vi "Save_Trav_setup.vi"(0 "Work in Tunnel Coordinates?":T1, 1 "Trav Table":T2[](array[typedef]) {"Row Duration (mins)" format="%#.1f"; "Row No" min=0; "Trace Gas Concentration (%)" min=0.0 format="%#.2f"; "Emission Rate (l/min)" format="%#.2f"; "Tunnel Speed" format="%#.2f"; "Start X" format="%#.2f"; "Start Y" format="%#.2f"; "Start Z" format="%#.2f"; "End X" format="%#.2f"; "End Y" format="%#.2f"; "End Z" format="%#.2f"; "Averaging time (min)" min=0.0 format="%#.1f"}, 3 "Jump Bad Positions":bool, 4 "Setup filename":path) -> (5 "Trav Table Out":T2[](array[typedef]) {"Row Duration (mins)" format="%#.1f"; "Row No" min=0; "Trace Gas Concentration (%)" min=0.0 format="%#.2f"; "Emission Rate (l/min)" format="%#.2f"; "Tunnel Speed" format="%#.2f"; "Start X" format="%#.2f"; "Start Y" format="%#.2f"; "Start Z" format="%#.2f"; "End X" format="%#.2f"; "End Y" format="%#.2f"; "End Z" format="%#.2f"; "Averaging time (min)" min=0.0 format="%#.1f"})   [LabVIEW 2010]
uses:
  Traverse_cluster.ctl
  Spacing.ctl
  Controls/Multi_run_mode.ctl
  Controls/Tunnel_Coordinates.ctl
  Globals/Constants_global.vi
panel:
  # "X           Y            Z"
  # "Start"
  # "End"
  # "X           Y            Z"
  # "Start"
  # "End"
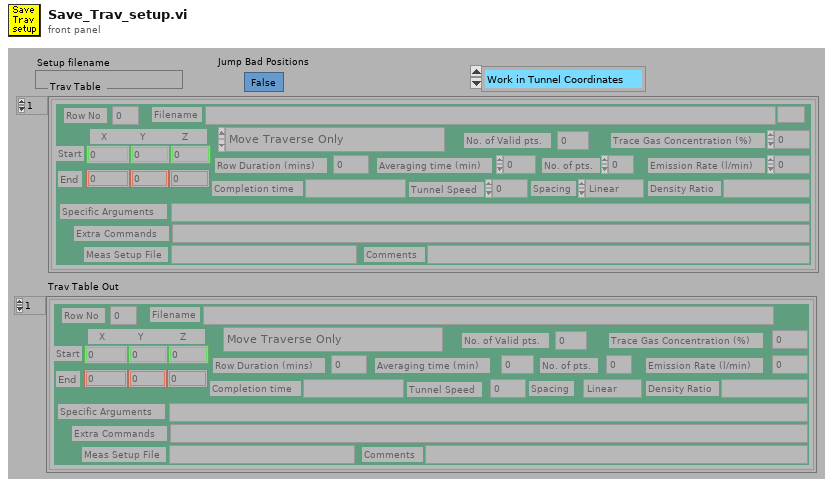
[diagram p1: front panel]
types:
  T1 = typedef "Tunnel_Coordinates.ctl" = enum16{"Work in Tunnel Coordinates", "Work in Model Coordinates"}
  T2 = typedef "Traverse_cluster.ctl" = cluster{"Start X":dbl, "Start Y":dbl, "Start Z":dbl, "End X":dbl, "End Y":dbl, "End Z":dbl, "No. of pts.":i32, "Spacing":T3, "Filename":path, "Tunnel Speed":dbl, "Averaging time (min)":dbl, "Extra Commands":string, "Specific Arguments":string, "Emission Rate (l/min)":dbl, "Trace Gas Concentration (%)":dbl, "Density Ratio":string, "Comments":string, "Row No":i32, "Row Type Selector":T4, "Completion time":string, "Row Duration (mins)":dbl, "No. of Valid pts.":i32, "Meas Setup File":string}
  T3 = typedef "Spacing.ctl" = enum16{"Linear", "Log", "Gauss", "Specified", "N/A"}
  T4 = typedef "Multi_run_mode.ctl" = enum16{"Move Traverse Only", "Set Tunnel Speed Only", "Set Source Only", "Set Measurement Conditions", "Single Measurement", "Vertical Profile", "Lateral Profile", "Longitudinal Profile", "Explore Volume", "Multi-Axis Profile", "Auto Calibrate", "Meas Fast FID Bkgnd", "Check Beam Power", "Scanning Valve Measurement", "Run VI Named:", "Set ADAM Ch", "Wait (minutes)", "Send Message", "Synchronize With:", "Fall Back to this Row", "Turn Off Row Repeating", "Blank Row"}
  T5 = enum16{"All Channel Names", "Valid Channel Names"}
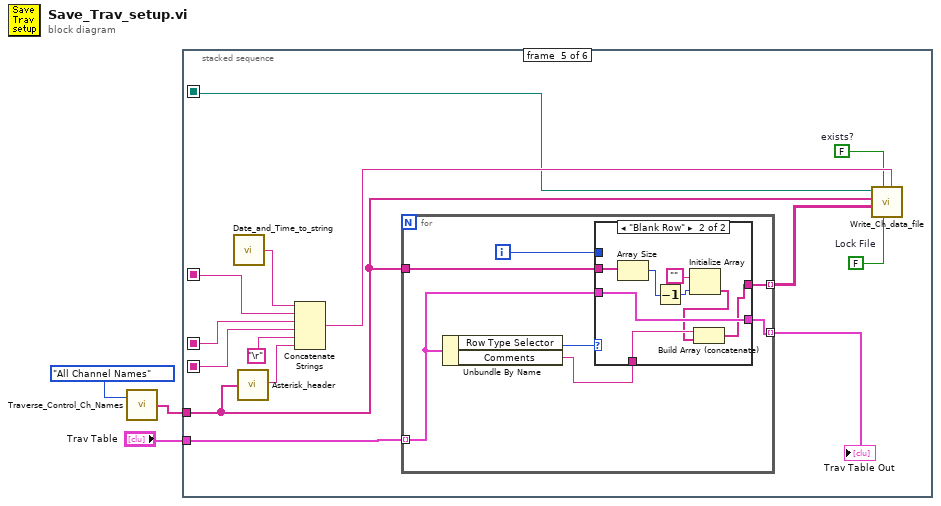
[diagram p0: block diagram]
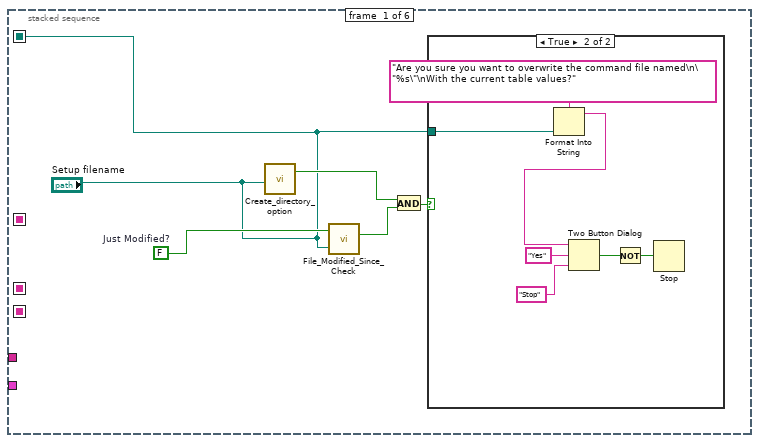
[diagram p2: hidden frame]
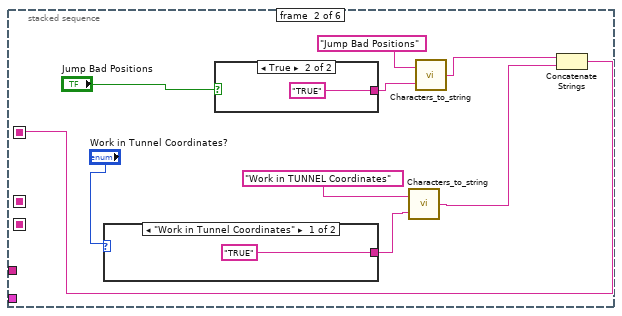
[diagram p4: hidden frame]
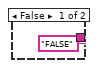
[diagram p5: hidden frame]
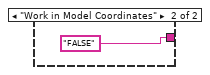
[diagram p6: hidden frame]
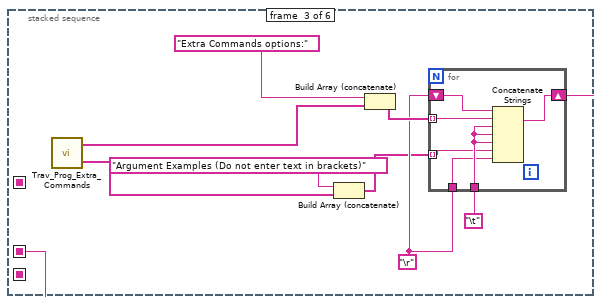
[diagram p7: hidden frame]
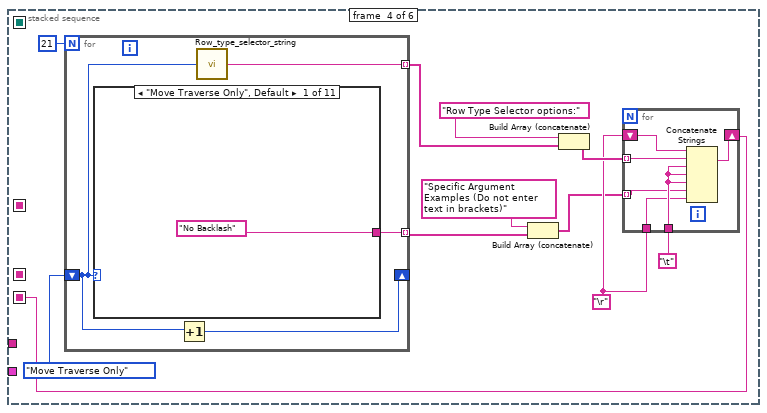
[diagram p8: hidden frame]
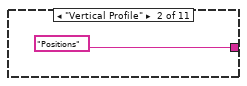
[diagram p9: hidden frame]
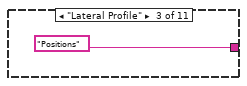
[diagram p10: hidden frame]
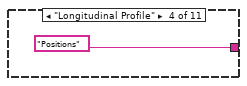
[diagram p11: hidden frame]
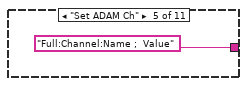
[diagram p12: hidden frame]
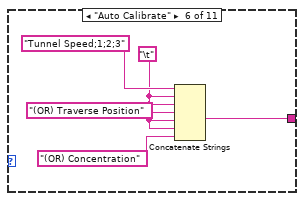
[diagram p13: hidden frame]
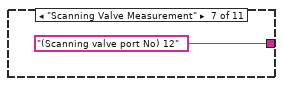
[diagram p14: hidden frame]
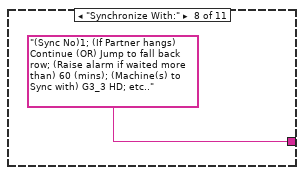
[diagram p15: hidden frame]
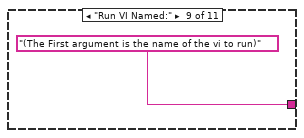
[diagram p16: hidden frame]
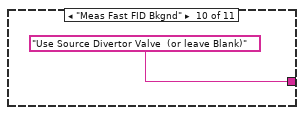
[diagram p17: hidden frame]
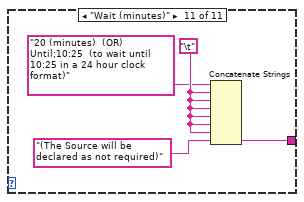
[diagram p18: hidden frame]
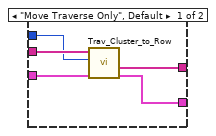
[diagram p19: hidden frame]
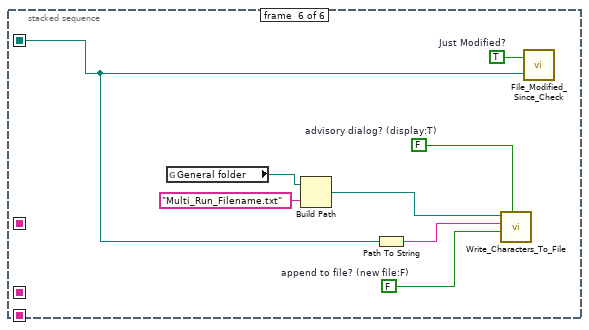
[diagram p20: hidden frame]
diagram:
  n1 = call "Traverse_Control_Ch_Names.vi"("Mode"=T5."All Channel Names") -> ("Channel names"=w3:string[])  [unwired: 1 in]
  n2 = stacked-sequence {
    seq-local: [_ w24 _ _ _ _] -> [_ _ _ _ w92 _]
    seq-local: [_ _ w35 _ _ _] -> [_ _ _ _ w94 _]
    seq-local: [_ _ _ w48 _ _] -> [_ _ _ _ w91 _]
    seq-local: ["Setup filename" _ _ _ _ _] -> [_ _ _ _ w84 w120]
    tunnel: w3 -> [_ _ _ _ w90 _]
    tunnel: "Trav Table" -> [_ _ _ _ w83 _]
    frame #0 {
      w5 = FALSE  # Just Modified?
      n3 = call "Create_directory_option.vi"("Filename"="Setup filename") -> ("Path is to existing File"=w7:bool)  [unwired: 1 out]
      n4 = call "File_Modified_Since_Check.vi"("Pathname"="Setup filename", "Just Modified?"=w5) -> ("Modified?"=w8:bool)
      n5 = And(x=w7, y=w8) -> (x .and. y?=w6:bool)
      n6 = case shown="True" w6 {
        tunnel: "Setup filename" -> [_ w15]
        frame False {
        }
        frame True {
          n7 = Format Into String(format string="Are you sure you want to overwrite the command file named\n\"%s\"\nWith the current table values?" ("Format String"), w15) -> (resulting string=w13:string)  [unwired: 2 in, 1 out]
          n8 = Two Button Dialog(message=w13, 1:"Stop" ("F button name (\"Cancel\")"), 2:"Yes" ("T button name (\"OK\")")) -> (T button?=w10:bool)
          n9 = Not(x=w10) -> (.not. x?=w9:bool)
          n10 = Stop(stop? (T)=w9) -> ()
        }
      }
    }
    frame #1 {
      n11 = case shown="\"Work in Tunnel Coordinates\"" "Work in Tunnel Coordinates?" {
        tunnel: ["TRUE" "FALSE" ("f")] -> w20
        frame "Work in Tunnel Coordinates" {
        }
        frame "Work in Model Coordinates" {
        }
      }
      n12 = case shown="True" "Jump Bad Positions" {
        tunnel: ["FALSE" ("f") "TRUE"] -> w18
        frame False {
        }
        frame True {
        }
      }
      n13 = call "Characters_to_string.vi"("Characters to write"=w20, "Label for characters"="Work in TUNNEL Coordinates") -> ("Output string"=w22:string)
      n14 = call "Characters_to_string.vi"("Characters to write"=w18, "Label for characters"="Jump Bad Positions") -> ("Output string"=w16:string)
      n15 = Concatenate Strings(w16, w22) -> (w24:string)
    }
    frame #2 {
      w36 = "\r"
      n16 = call "Trav_Prog_Extra_Commands.vi"() -> ("Extra Commands Array"=w33:string[], "Argument Examples"=w32:string[])  [unwired: 1 out]
      n17 = Build Array (concatenate)("Argument Examples (Do not enter text in brackets)" ("Substring"), w32) -> (w31:string[])
      n18 = Build Array (concatenate)("Extra Commands options:", w33) -> (w37:string[])
      n19 = for {
        shift-right: [w41] -> w35
        shift-left: w36 -> [w42]
        tunnel: w37 -> [w43] mode=indexing
        tunnel: w36 -> [w38]
        tunnel: w31 -> [w39] mode=indexing
        tunnel: "\t" -> [w40]
        n20 = Concatenate Strings(w42, w43, w40, w40, w40, w39, w38) -> (w41:string)
      }
    }
    frame #3 {
      w53 = "\r"
      n21 = for {
        N: 21 -> [_]
        shift-right: [w58] -> _
        shift-left: Multi_run_mode."Move Traverse Only" ("Mode") -> [w57]
        tunnel: [w56] -> w46 mode=indexing
        tunnel: [w55] -> w45 mode=indexing
        n22 = case shown="\"Move Traverse Only\", Default" w57 {
          tunnel: ["No Backlash" "Positions" "Positions" "Positions" "Full:Channel:Name ;  Value" w68 "(Scanning valve port No) 12" "(Sync No)1; (If Partner hangs) Continue (OR) Jump to fall back row; (Raise alarm if waited more than) 60 (mins); (Machine(s) to Sync with) G3_3 HD; etc.." "(The First argument is the name of the vi to run)" "Use Source Divertor Valve  (or leave Blank)" w76] -> w55
          frame "Move Traverse Only", Default {
          }
          frame "Vertical Profile" {
          }
          frame "Lateral Profile" {
          }
          frame "Longitudinal Profile" {
          }
          frame "Set ADAM Ch" {
          }
          frame "Auto Calibrate" {
            w65 = "\t"
            n23 = Concatenate Strings("Tunnel Speed;1;2;3", w65, w65, "(OR) Traverse Position", w65, w65, "(OR) Concentration") -> (w68:string)
          }
          frame "Scanning Valve Measurement" {
          }
          frame "Synchronize With:" {
          }
          frame "Run VI Named:" {
          }
          frame "Meas Fast FID Bkgnd" {
          }
          frame "Wait (minutes)" {
            w74 = "\t"
            n24 = Concatenate Strings("20 (minutes)  (OR) Until;10:25  (to wait until 10:25 in a 24 hour clock format)" ("Substring"), w74, w74, w74, w74, w74, w74, "(The Source will be declared as not required)") -> (w76:string)
          }
        }
        n25 = Increment(x=w57) -> (x+1=w58:T4)
        n26 = call "Row_type_selector_string.vi"("Mode"=w57) -> ("Output string"=w56:string)
      }
      n27 = Build Array (concatenate)("Specific Argument Examples (Do not enter text in brackets)" ("Substring"), w45) -> (w51:string[])
      n28 = Build Array (concatenate)("Row Type Selector options:", w46) -> (w54:string[])
      n29 = for {
        shift-right: [w80] -> w48
        shift-left: w53 -> [w81]
        tunnel: w54 -> [w82] mode=indexing
        tunnel: w53 -> [w77]
        tunnel: w51 -> [w78] mode=indexing
        tunnel: "\t" -> [w79]
        n30 = Concatenate Strings(w81, w82, w79, w79, w79, w78, w77) -> (w80:string)
      }
    }
    frame #4 {
      w85 = FALSE  # Lock File
      w95 = FALSE  # exists?
      n31 = call "Date_and_Time_to_string.vi"() -> ("Date and time (spreadsheet)"=w93:string)
      n32 = call "Asterisk_header.vi"("Channel names"=w90) -> ("Header string"=w86:string)
      n33 = Concatenate Strings(w93, w92, w94, w91, "\r", w86) -> (w96:string)
      n34 = for {
        tunnel: w90 -> [w103]
        tunnel: w83 -> [w99] mode=indexing
        tunnel: [w102] -> w89 mode=indexing
        tunnel: [w101] -> w88 mode=indexing
        i -> [w100]
        n35 = Unbundle By Name(w99) -> ("Row Type Selector"=w98:T4, "Comments"=w97:string)
        n36 = case shown="\"Blank Row\"" w98 {
          tunnel: w103 -> [w108 w115]
          tunnel: [w107 w109] -> w102
          tunnel: [w106 w116] -> w101
          tunnel: w100 -> [w105 _]
          tunnel: w99 -> [w104 w116]
          tunnel: w97 -> [_ w111]
          frame "Move Traverse Only", Default {
            n37 = call "Trav_Cluster_to_Row.vi"("Traverse line in"=w104, "Row Number"=w105, "Channel names"=w108) -> ("Traverse line Out"=w106:T2, "Channel Values Out"=w107:string[])  [unwired: 3 out]
          }
          frame "Blank Row" {
            n38 = Array Size(array=w115) -> (size(s)=w113:i32)
            n39 = Decrement(x=w113) -> (x-1=w112:i32)
            n40 = Initialize Array("", w112) -> (w110:string[])
            n41 = Build Array (concatenate)(w111, w110) -> (w109:string[])
          }
        }
      }
      "Trav Table Out" <- w88
      n42 = call "Write_Ch_data_file.vi"("Header string"=w96, "Lock File"=w85, "exists?"=w95, "Channel Values"=w89, "Channel names"=w90, "Filename"=w84) -> ()  [unwired: 2 in, 4 out]
    }
    frame #5 {
      w117 = FALSE  # append to file? (new file:F)
      w118 = FALSE  # advisory dialog? (display:T)
      w124 = TRUE  # Just Modified?
      n43 = global read "Constants_global.vi" "General folder"() -> (w123:path)
      n44 = Build Path(base path=w123, name or relative path="Multi_Run_Filename.txt") -> (appended path=w121:path)
      n45 = Path To String(path=w120) -> (string=w119:string)
      n46 = call "Write_Characters_To_File.vi"("file path (dialog if empty)"=w121, "advisory dialog? (display:T)"=w118, "character string"=w119, "append to file? (new file:F)"=w117) -> ()  [unwired: 1 in, 4 out]
      n47 = call "File_Modified_Since_Check.vi"("Pathname"=w120, "Just Modified?"=w124) -> ()  [unwired: 1 out]
    }
  }
